vi "DiffDriveTrainSim_SetPose.vi"(10 "Pose":T5={"TRANSLATION"={"X"=0.0, "Y"=0.0}, "ROTATION"={"VALUE"=0.0, "COS"=1.0, "SIN"=0.0}} {"ROTATION"."SIN" format="%13.4f"; "ROTATION"."COS" format="%13.4f"; "ROTATION"."VALUE" format="%13.4f"; "TRANSLATION"."Y" format="%14.3f"; "TRANSLATION"."X" format="%14.3f"}, 11 "in DiffDriveTrainSim":T1 {"m_Motor"."Jr_KgM2" format="%13.5p"; "m_Motor"."L_H" format="%13.5p"; "m_Motor"."Kt_NMPerAmp" format="%13.5p"; "m_Motor"."KvINV_RadPerSecPerVolt" format="%13.5p"; "m_Motor"."R_Ohms" format="%13.5p"; "m_Motor"."FreeSpeed_RadPerSec" format="%13.5p"; "m_Motor"."FreeCurrent_Amps" format="%13.5p"; "m_Motor"."StallCurrent_Amps" format="%13.5p"; "m_Motor"."StallTorque_NM" format="%13.5p"; "m_Motor"."nominalVoltage_Volts" format="%13.5p"}) -> (3 "out DiffDriveTrainSim":T1 {"m_Motor"."Jr_KgM2" format="%13.5p"; "m_Motor"."L_H" format="%13.5p"; "m_Motor"."Kt_NMPerAmp" format="%13.5p"; "m_Motor"."KvINV_RadPerSecPerVolt" format="%13.5p"; "m_Motor"."R_Ohms" format="%13.5p"; "m_Motor"."FreeSpeed_RadPerSec" format="%13.5p"; "m_Motor"."FreeCurrent_Amps" format="%13.5p"; "m_Motor"."StallCurrent_Amps" format="%13.5p"; "m_Motor"."StallTorque_NM" format="%13.5p"; "m_Motor"."nominalVoltage_Volts" format="%13.5p"})   [LabVIEW 2019, in "Trajectory_Library.lvlib"]
doc: "Sets the system pose.\n \nInputs:\n - DiffDriveTraimSim -- Data cluster\n - pose -- The pose.\n\nOutputs:\n - OutDiffDriveTraimSim -- Updated data cluster."
uses:
  Trajectory_Library.lvlib
  DIFF_DRIVE_TRAIN_SIM.ctl
  LINEAR_SYSTEM.ctl
  <vilib>/Analysis/Matrix/Datatypes/RealMatrix.ctl
  DCMOTOR.CTL
  POSE2D.ctl
  TRANSLATION2D.ctl
  ROTATION2D.ctl
  DIFF_DRIVE_TRAIN_SIM_STATE_ENUM.ctl
  <vilib>/Analysis/Matrix/NI_Matrix.lvlib
panel:
  # "<States, 1>"
  # "<Outputs, 1>"
  # "<Inputs, 1>"
  # "<Outputs, 1>"
  # "<States,States>"
  # "<States,Inputs>"
  # "<Outputs,States>"
  # "<Outputs,Inputs>"
  # "<States, 1>"
  # "<Outputs, 1>"
  # "<Inputs, 1>"
  # "<Outputs, 1>"
  # "<States,States>"
  # "<States,Inputs>"
  # "<Outputs,States>"
  # "<Outputs,Inputs>"
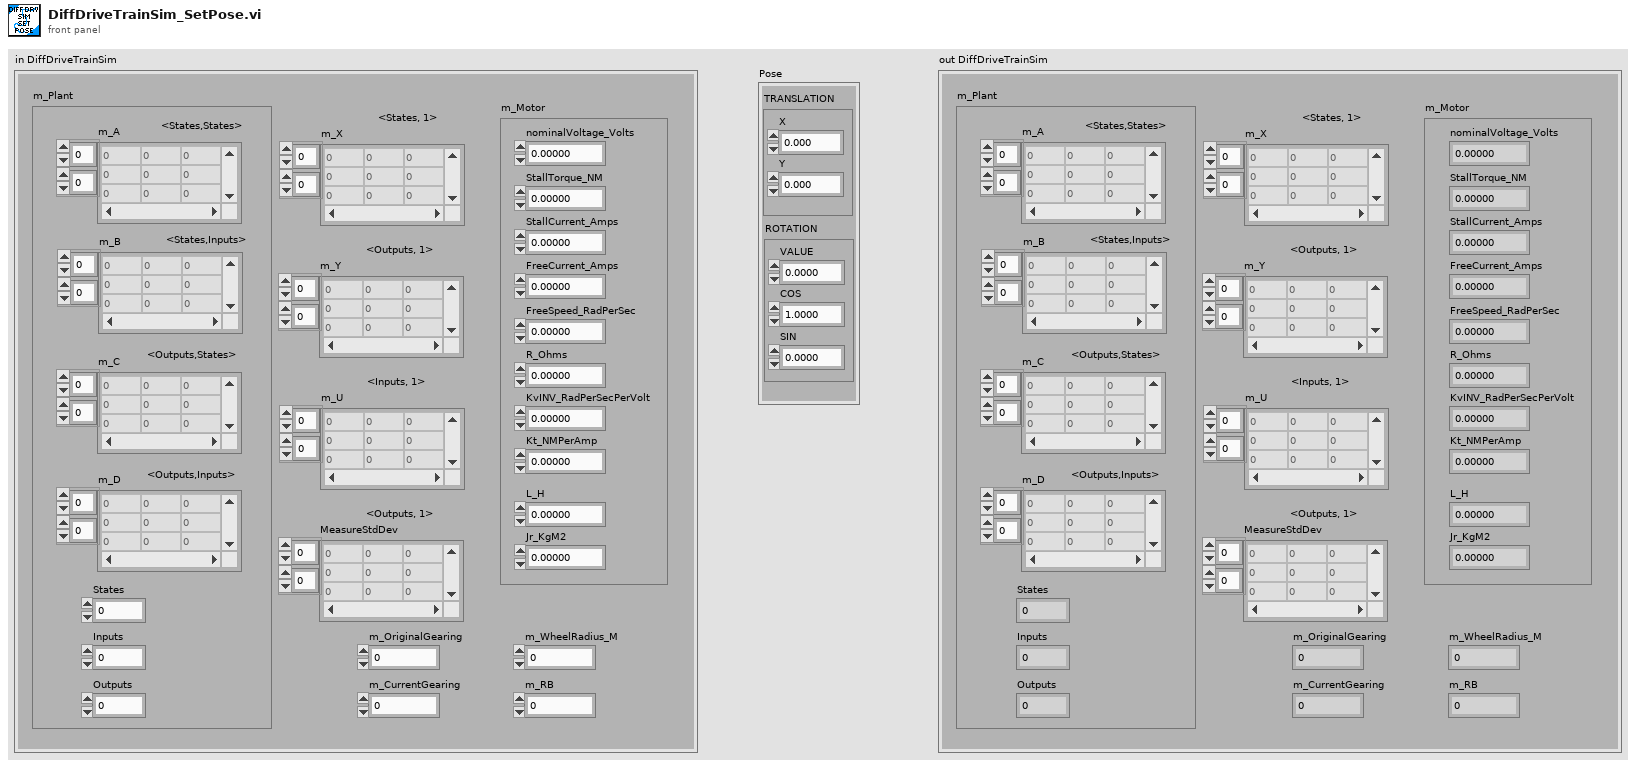
[diagram p1: front panel]
types:
  T1 = typedef "Trajectory_Library.lvlib/DIFF_DRIVE_TRAIN_SIM.ctl" = cluster{"m_Plant":T2, "m_X":T3, "m_Y":T3, "m_U":T3, "MeasureStdDev":T3, "m_Motor":T4, "m_OriginalGearing":dbl, "m_CurrentGearing":dbl, "m_WheelRadius_M":dbl, "m_RB":dbl}
  T2 = typedef "Trajectory_Library.lvlib/LINEAR_SYSTEM.ctl" = cluster{"m_A":T3, "m_B":T3, "m_C":T3, "m_D":T3, "States":i32, "Inputs":i32, "Outputs":i32}
  T3 = typedef "NI_Matrix.lvlib/RealMatrix.ctl" = dbl[][]
  T4 = typedef "Trajectory_Library.lvlib/DCMOTOR.CTL" = cluster{"nominalVoltage_Volts":dbl, "StallTorque_NM":dbl, "StallCurrent_Amps":dbl, "FreeCurrent_Amps":dbl, "FreeSpeed_RadPerSec":dbl, "R_Ohms":dbl, "KvINV_RadPerSecPerVolt":dbl, "Kt_NMPerAmp":dbl, "L_H":dbl, "Jr_KgM2":dbl}
  T5 = typedef "Trajectory_Library.lvlib/POSE2D.ctl" = cluster{"TRANSLATION":T6, "ROTATION":T7}
  T6 = typedef "Trajectory_Library.lvlib/TRANSLATION2D.ctl" = cluster{"X":dbl, "Y":dbl}
  T7 = typedef "Trajectory_Library.lvlib/ROTATION2D.ctl" = cluster{"VALUE":dbl, "COS":dbl, "SIN":dbl}
  T8 = typedef "Trajectory_Library.lvlib/DIFF_DRIVE_TRAIN_SIM_STATE_ENUM.ctl" = enum16{"X_POS", "Y_POS", "HEADING", "LEFT_VEL", "RIGHT_VEL", "LEFT_DIST", "RIGHT_DIST"}
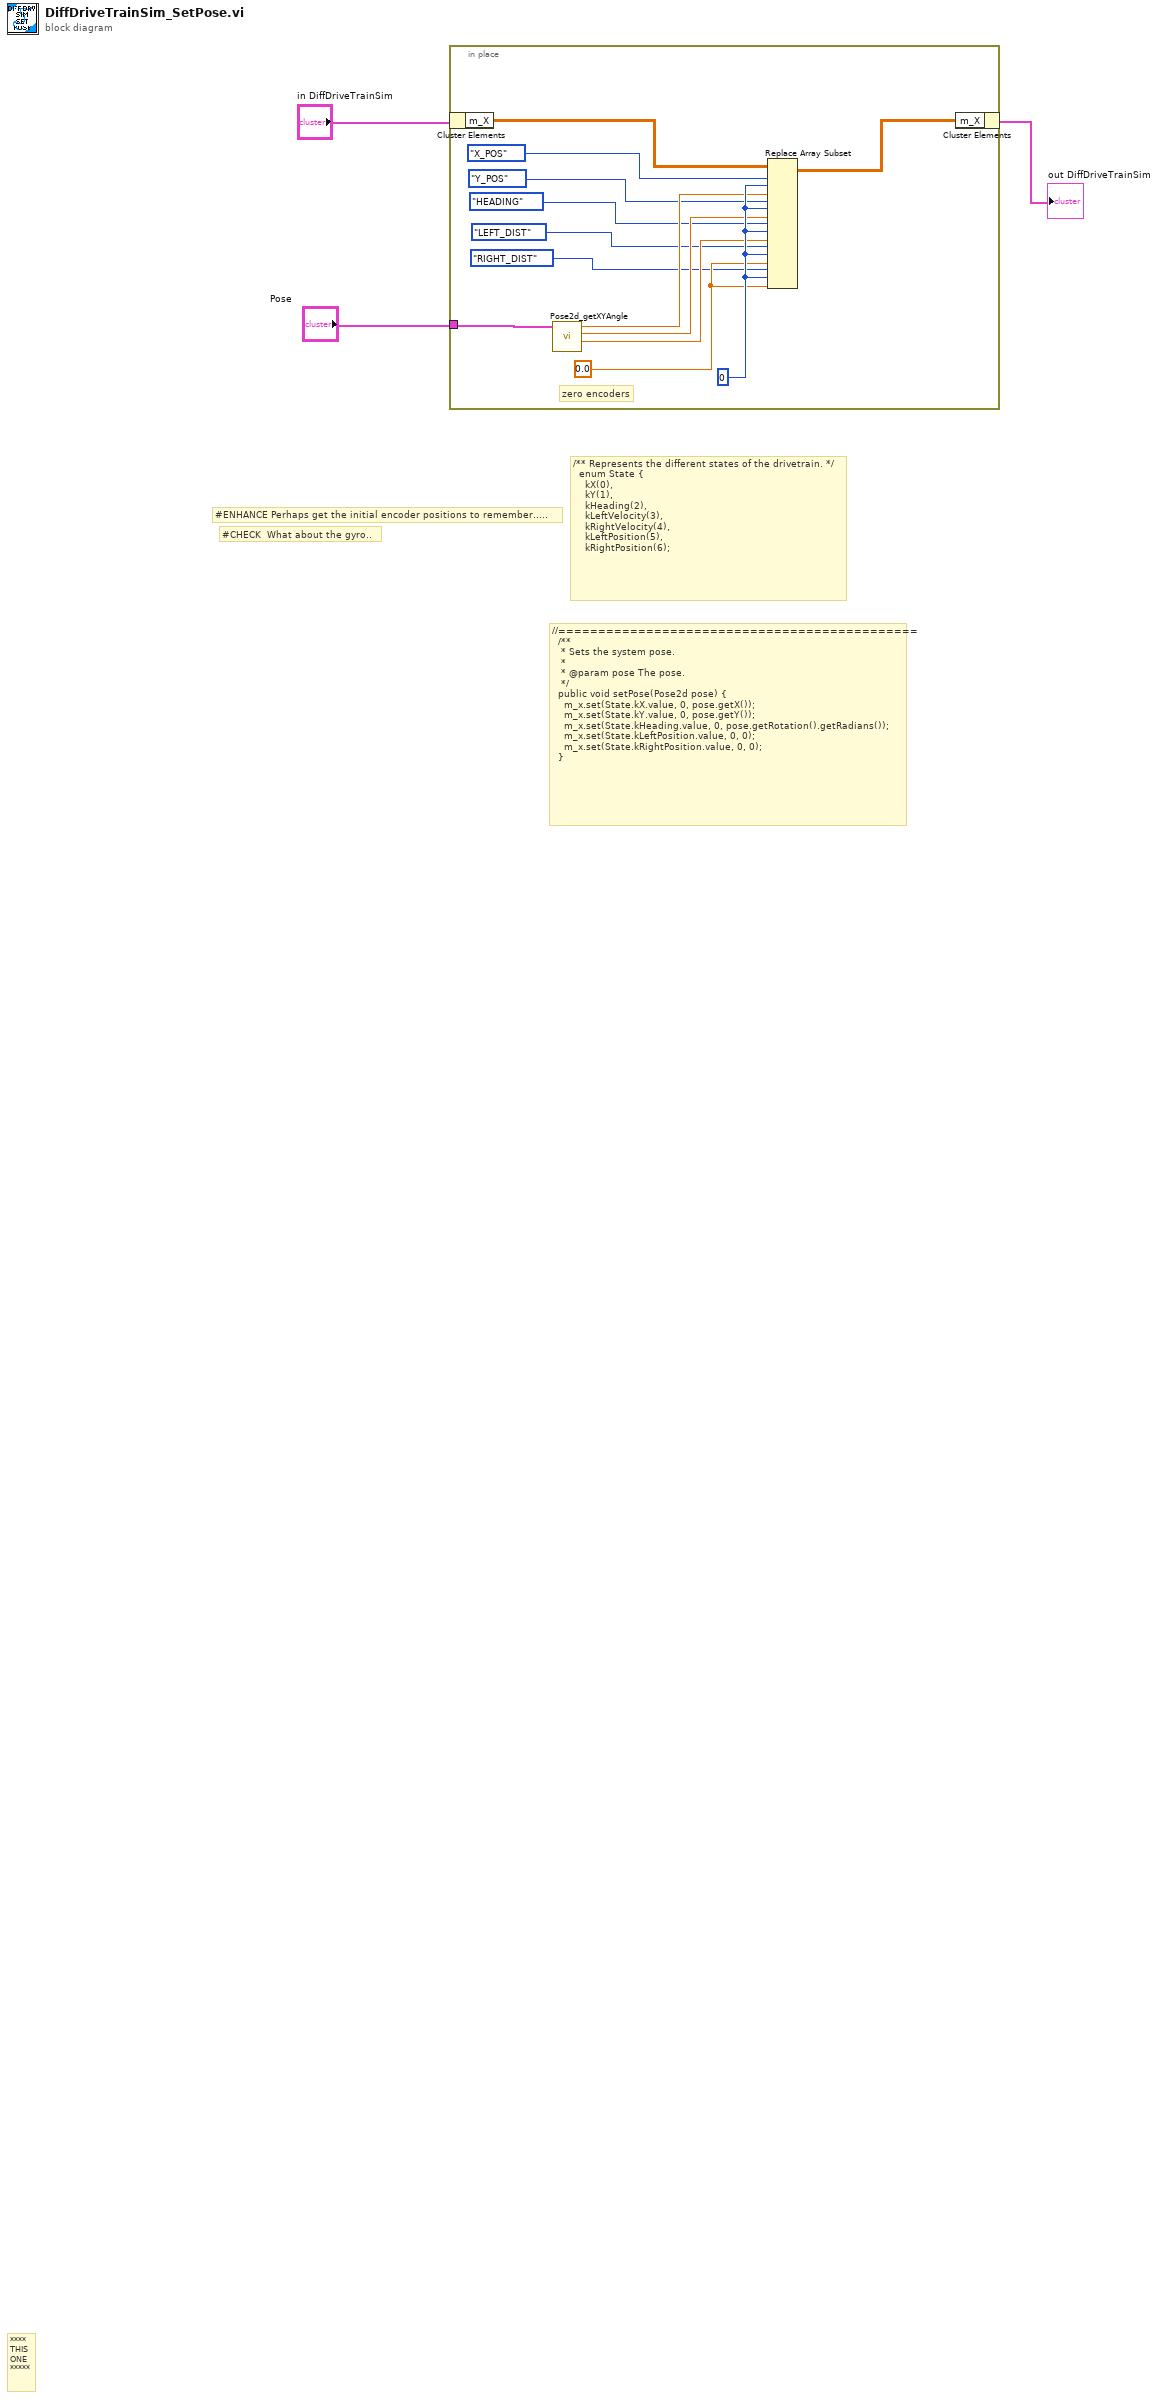
[diagram p0: block diagram]
diagram:
  # "#CHECK  What about the gyro.."
  # "#ENHANCE Perhaps get the initial encoder positions to remember....."
  # "//=============================================\n  /**\n   * Sets the system pose.\n   *\n   * @param pose The pose.\n   */\n  public void setPose(Pose2d pose) {\n    m_x.set(State.kX.value, 0, pose.getX());\n    m_x.set(State.kY.value, 0, pose.getY());\n    m_x.set(State.kHeading.value, 0, pose.getRotation().getRadians());\n    m_x.set(State.kLeftPosition.value, 0, 0);\n    m_x.set(State.kRightPosition.value, 0, 0);\n  }"
  # "/** Represents the different states of the drivetrain. */\n  enum State {\n    kX(0),\n    kY(1),\n    kHeading(2),\n    kLeftVelocity(3),\n    kRightVelocity(4),\n    kLeftPosition(5),\n    kRightPosition(6);"
  # "****\nTHIS\nONE\n*****"
  n1 = in-place {
    in-place-border: "Pose" -> [w16]
    w10 = 0.0 ("new element/submatrix")
    w14 = 0 ("index (col)")
    # "zero encoders"
    n2 = in-place-cluster #1("in DiffDriveTrainSim") -> ("m_X"=w15:T3)
    n3 = call "Pose2d_getXYAngle.vi"("in POSE"=w16) -> ("Angle"=w11:dbl, "Y"=w12:dbl, "X"=w13:dbl)  [unwired: 8 in]
    n4 = Replace Array Subset(array=w15, new element #1=w13, index (row) #1=DIFF_DRIVE_TRAIN_SIM_STATE_ENUM."X_POS" ("DIFF_DRIVE_TRAIN_SIM_STATE"), index (col) #1=w14, new element #2=w12, index (row) #2=DIFF_DRIVE_TRAIN_SIM_STATE_ENUM."Y_POS" ("DIFF_DRIVE_TRAIN_SIM_STATE"), index (col) #2=w14, new element #3=w11, index (row) #3=DIFF_DRIVE_TRAIN_SIM_STATE_ENUM."HEADING" ("DIFF_DRIVE_TRAIN_SIM_STATE"), index (col) #3=w14, new element #4=w10, index (row) #4=DIFF_DRIVE_TRAIN_SIM_STATE_ENUM."LEFT_DIST" ("DIFF_DRIVE_TRAIN_SIM_STATE"), index (col) #4=w14, new element #5=w10, index (row) #5=DIFF_DRIVE_TRAIN_SIM_STATE_ENUM."RIGHT_DIST" ("DIFF_DRIVE_TRAIN_SIM_STATE"), index (col) #5=w14) -> (w9:T3)
    n5 = in-place-cluster #1("m_X"=w9) -> (→"out DiffDriveTrainSim":T1)
  }
